vi "CoolProp_HAProp_SI_V9.0.vi"(4 "Value2":dbl, 5 "Value1":dbl, 6 "Humidity parameter":T1(ring), 7 "Dry bulb temperature of moist air":enum16{"T [K]"}(ring), 8 "error in (no error)":errorcluster, 9 "Output":string, 11 "path in":path) -> (0 "error out":errorcluster, 2 "error_message":string, 3 "Return Value":dbl)   [LabVIEW 2009]
panel:
  in  "Absolute pressure of moist air":enum16{"P [Pa]"}(ring)
  in  "Value3":dbl
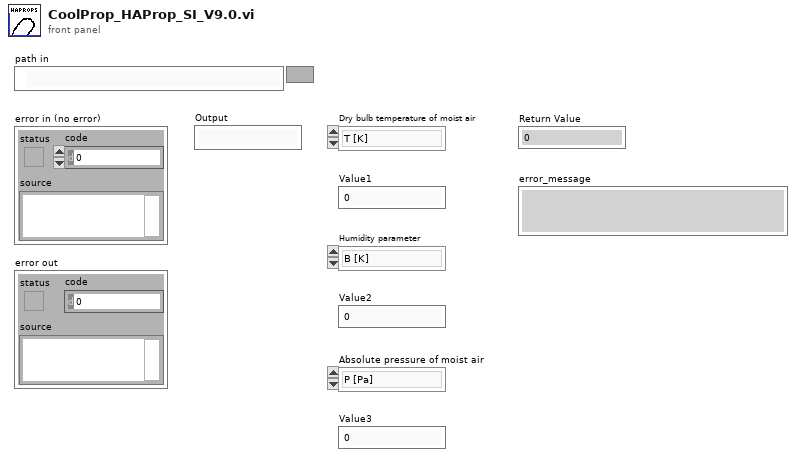
[diagram p1: front panel]
types:
  T1 = enum16{"B [K]", "D [K]", "R [-]", "W [kg wv/kg da]"}
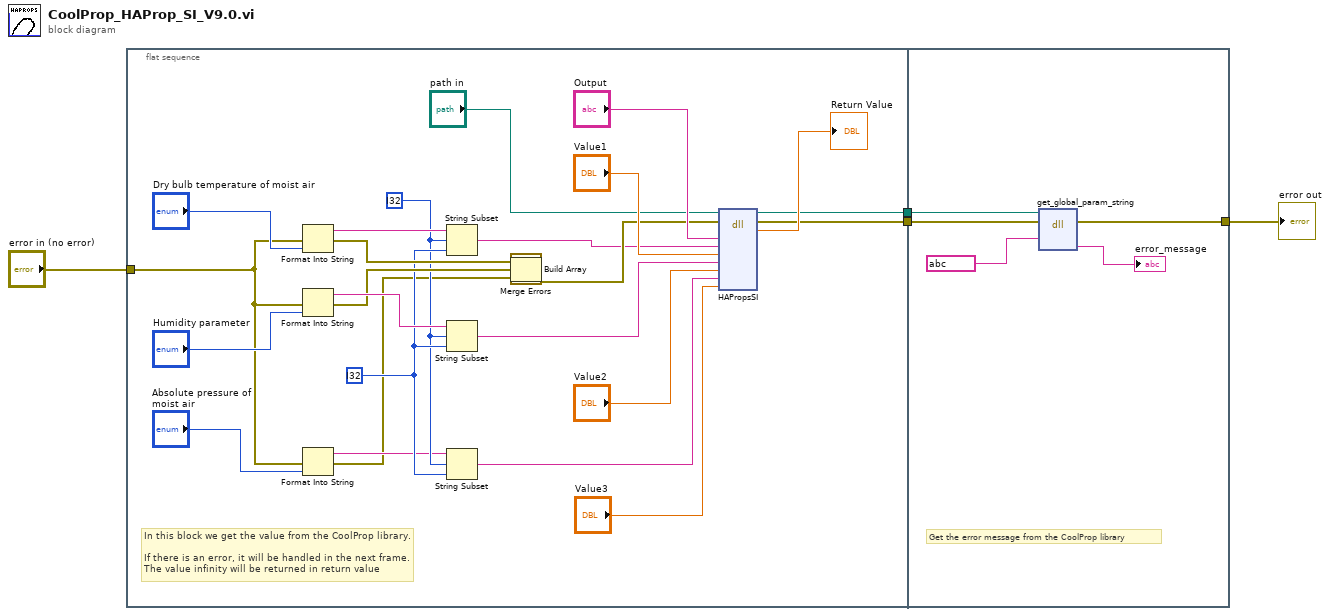
[diagram p0: block diagram]
diagram:
  n1 = flat-sequence {
    tunnel: "error in (no error)" -> [w9]
    tunnel: [w16] -> w3
    tunnel: [w15] -> w1
    tunnel: w3 -> [w32]
    tunnel: [w31] -> w2
    tunnel: w1 -> [w30]
    frame #0 {
      w12 = i32 ? ("length (rest)")
      w11 = i32 ? ("offset (0)")
      # "In this block we get the value from the CoolProp library.\n\nIf there is an error, it will be handled in the next frame.\nThe value infinity will be returned in return value"
      n2 = Format Into String(error in=w9, "Dry bulb temperature of moist air") -> (resulting string=w25:string, error out=w23:errorcluster)  [unwired: 2 in]
      n3 = Format Into String(error in=w9, "Humidity parameter") -> (resulting string=w24:string, error out=w22:errorcluster)  [unwired: 2 in]
      n4 = Format Into String(error in=w9, "Absolute pressure of moist air") -> (resulting string=w8:string, error out=w6:errorcluster)  [unwired: 2 in]
      n5 = String Subset(string=w25, offset (0)=w11, length (rest)=w12) -> (substring=w18:string)
      n6 = String Subset(string=w24, offset (0)=w11, length (rest)=w12) -> (substring=w17:string)
      n7 = String Subset(string=w8, offset (0)=w11, length (rest)=w12) -> (substring=w7:string)
      n8 = Build Array(w23, w22, w6) -> (w5:errorcluster[])
      n9 = call <vilib>:"Merge Errors.vi"("error array in"=w5) -> ("error out"=w21:errorcluster)  [unwired: 6 in]
      n10 = dll-call lib="C:/Program Files (x86)/National Instruments/LabVIEW 2015/user.lib/CoolProp.dll" fn="HAPropsSI"(path in="path in", error in=w21, "Output"="Output", "Input1"=w18, "Value1"="Value1", "Input2"=w17, "Value2"="Value2", "Input3"=w7, "Value3"="Value3") -> (path out=w15:path, error out=w16:errorcluster, "OutputValue"=→"Return Value":dbl)  [unwired: 8 in]
    }
    frame #1 {
      # "Get the error message from the CoolProp library"
      n11 = dll-call lib="C:/Program Files (x86)/National Instruments/LabVIEW 2011/user.lib/CoolProp.dll" fn="get_global_param_string"(path in=w30, error in=w32, "param"=string ?) -> (error out=w31:errorcluster, "error_message"=→"error_message":string)  [unwired: 2 in, 3 out]
    }
  }
  "error out" <- w2
